vi "FP handling.vi"(6 "Set Modal?":bool, 7 "Mode":T3=enum."Restore Properties", 8 "error in (no error)":errorcluster, 10 "Properties Input":T1, 11 "VI in":refnum<vi>) -> (0 "error out":errorcluster, 2 "Retrieved Properties":T1, 3 "VI out":refnum<vi>)   [LabVIEW 2020]
uses:
  <vilib>/Utility/miscctls.llb/LVRectTypeDef.ctl
  FP UserInterface Properties--cluster.ctl
  FP handling mode selection--enum.ctl
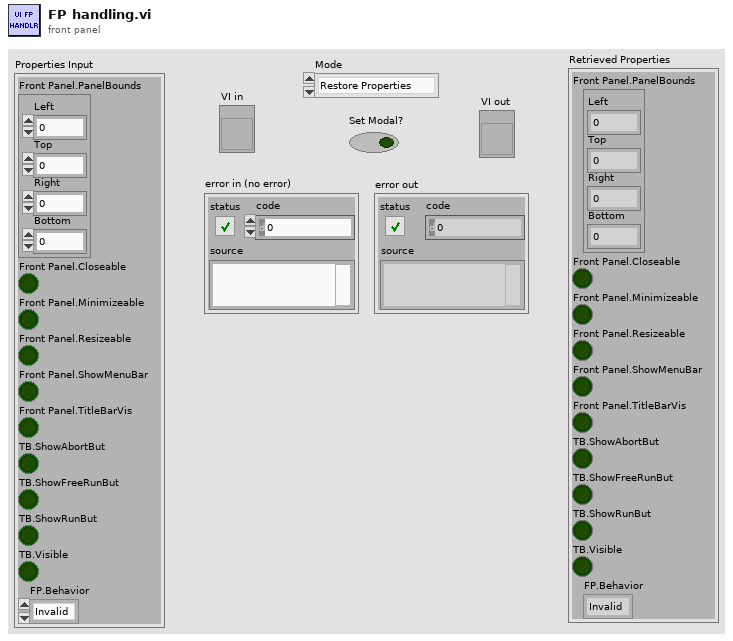
[diagram p1: front panel]
types:
  T1 = typedef "FP UserInterface Properties--cluster.ctl" = cluster{"Front Panel.PanelBounds":T2, "Front Panel.Closeable":bool, "Front Panel.Minimizeable":bool, "Front Panel.Resizeable":bool, "Front Panel.ShowMenuBar":bool, "Front Panel.TitleBarVis":bool, "TB.ShowAbortBut":bool, "TB.ShowFreeRunBut":bool, "TB.ShowRunBut":bool, "TB.Visible":bool, "FP.Behavior":enum32{"Invalid", "Default", "Floating", "Floating/Auto-Hide", "Modal"}}
  T2 = typedef "LVRectTypeDef.ctl" = cluster{"Left":i16, "Top":i16, "Right":i16, "Bottom":i16}
  T3 = typedef "FP handling mode selection--enum.ctl" = enum16{"Get Properties", "Restore Properties", "Set Full TouchScreen", "Properties Input"}
  T4 = enum32{"Invalid", "Default", "Floating", "Floating/Auto-Hide", "Modal"}
  T5 = cluster{"Front Panel Window:Panel Bounds":T2, "Front Panel.Closeable":bool, "Front Panel.Closeable":bool, "Front Panel.Closeable":bool, "Front Panel.Closeable":bool, "Front Panel.Closeable":bool, "Front Panel.Closeable":bool, "Front Panel.Closeable":bool, "Front Panel.Closeable":bool, "Front Panel.Closeable":bool, "Front Panel Window:Behavior":enum32{"Invalid", "Default", "Floating", "Floating/Auto-Hide", "Modal"}}
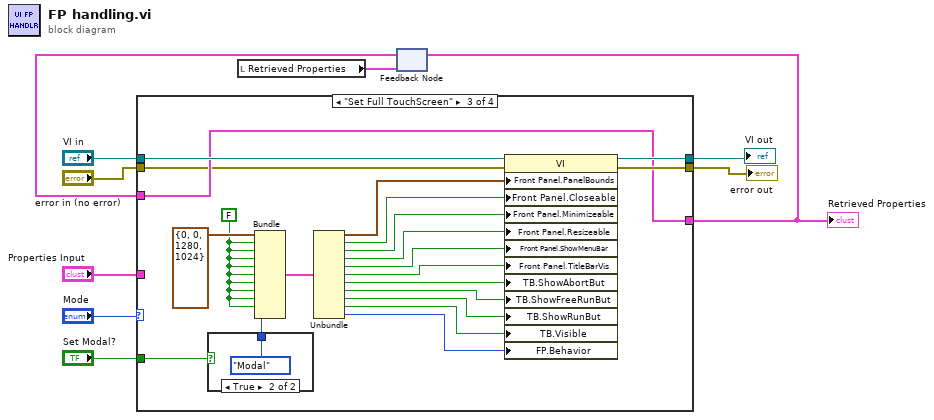
[diagram p0: block diagram]
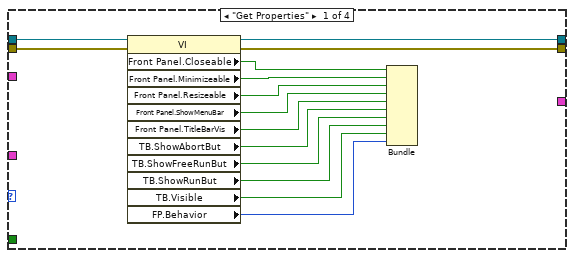
[diagram p2: hidden frame]
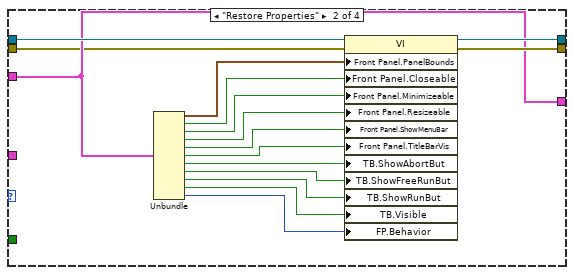
[diagram p3: hidden frame]
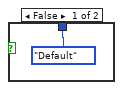
[diagram p4: hidden frame]
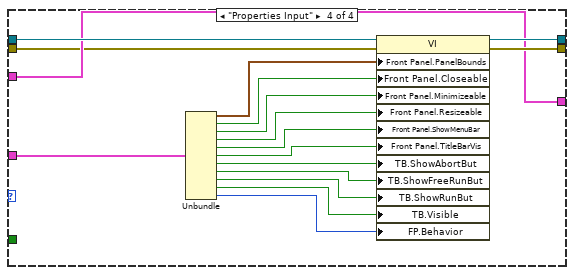
[diagram p5: hidden frame]
diagram:
  n1 = local read "Retrieved Properties"() -> (w3:T1)
  n2 = feedback #1(w3) -> (w6:T1)
  n3 = case shown="\"Set Full TouchScreen\"" "Mode" {
    tunnel: "VI in" -> [w14 w28 w49 w68]
    tunnel: [w13 w27 w48 w67] -> w8
    tunnel: [w12 w29 w50 w69] -> w9
    tunnel: [_ w26 w47 w66] -> w7
    tunnel: w6 -> [_ w26 w47 w66]
    tunnel: "error in (no error)" -> [w11 w25 w46 w65]
    tunnel: "Set Modal?" -> [_ _ w41 _]
    tunnel: "Properties Input" -> [_ _ _ w64]
    frame "Get Properties" {
      n4 = property class="VI"(reference=w14, error in=w11) -> (reference out=w12:refnum<vi>, error out=w13:errorcluster, "Front Panel.Closeable"=w22:bool, "Front Panel.Minimizeable"=w15:bool, "Front Panel.Resizeable"=w16:bool, "Front Panel.ShowMenuBar"=w17:bool, "Front Panel.TitleBarVis"=w18:bool, "TB.ShowAbortBut"=w19:bool, "TB.ShowFreeRunBut"=w20:bool, "TB.ShowRunBut"=w24:bool, "TB.Visible"=w21:bool, "FP.Behavior"=w23:T4)
      n5 = Bundle("Front Panel.Closeable"=w22, "Front Panel.Minimizeable"=w15, "Front Panel.Resizeable"=w16, "Front Panel.ShowMenuBar"=w17, "Front Panel.TitleBarVis"=w18, "TB.ShowAbortBut"=w19, "TB.ShowFreeRunBut"=w20, "TB.ShowRunBut"=w24, "TB.Visible"=w21, "FP.Behavior"=w23) -> ()  [unwired: 1 in, 1 out]
    }
    frame "Restore Properties" {
      n6 = Unbundle(w26) -> ("Front Panel.PanelBounds"=w30:T2, "Front Panel.Closeable"=w31:bool, "Front Panel.Minimizeable"=w32:bool, "Front Panel.Resizeable"=w33:bool, "Front Panel.ShowMenuBar"=w34:bool, "Front Panel.TitleBarVis"=w35:bool, "TB.ShowAbortBut"=w36:bool, "TB.ShowFreeRunBut"=w37:bool, "TB.ShowRunBut"=w38:bool, "TB.Visible"=w39:bool, "FP.Behavior"=w40:T4)
      n7 = property class="VI"(reference=w28, error in=w25, "Front Panel.PanelBounds"=w30, "Front Panel.Closeable"=w31, "Front Panel.Minimizeable"=w32, "Front Panel.Resizeable"=w33, "Front Panel.ShowMenuBar"=w34, "Front Panel.TitleBarVis"=w35, "TB.ShowAbortBut"=w36, "TB.ShowFreeRunBut"=w37, "TB.ShowRunBut"=w38, "TB.Visible"=w39, "FP.Behavior"=w40) -> (reference out=w29:refnum<vi>, error out=w27:errorcluster)
    }
    frame "Set Full TouchScreen" {
      w44 = FALSE ("Front Panel.Closeable")
      n8 = case shown="True" w41 {
        tunnel: [T4."Default" ("Front Panel Window:Behavior") T4."Modal" ("Front Panel Window:Behavior")] -> w43
        frame False {
        }
        frame True {
        }
      }
      n9 = Bundle("Front Panel Window:Panel Bounds"=T2 {"Left"=0, "Top"=0, "Right"=1280, "Bottom"=1024}, "Front Panel.Closeable"=w44, "Front Panel.Closeable"=w44, "Front Panel.Closeable"=w44, "Front Panel.Closeable"=w44, "Front Panel.Closeable"=w44, "Front Panel.Closeable"=w44, "Front Panel.Closeable"=w44, "Front Panel.Closeable"=w44, "Front Panel.Closeable"=w44, "Front Panel Window:Behavior"=w43) -> (w42:T5)  [unwired: 1 in]
      n10 = Unbundle(w42) -> ("Front Panel Window:Panel Bounds"=w51:T2, "Front Panel.Closeable"=w52:bool, "Front Panel.Closeable"=w53:bool, "Front Panel.Closeable"=w54:bool, "Front Panel.Closeable"=w55:bool, "Front Panel.Closeable"=w56:bool, "Front Panel.Closeable"=w57:bool, "Front Panel.Closeable"=w58:bool, "Front Panel.Closeable"=w59:bool, "Front Panel.Closeable"=w60:bool, "Front Panel Window:Behavior"=w61:T4)
      n11 = property class="VI"(reference=w49, error in=w46, "Front Panel.PanelBounds"=w51, "Front Panel.Closeable"=w52, "Front Panel.Minimizeable"=w53, "Front Panel.Resizeable"=w54, "Front Panel.ShowMenuBar"=w55, "Front Panel.TitleBarVis"=w56, "TB.ShowAbortBut"=w57, "TB.ShowFreeRunBut"=w58, "TB.ShowRunBut"=w59, "TB.Visible"=w60, "FP.Behavior"=w61) -> (reference out=w50:refnum<vi>, error out=w48:errorcluster)
    }
    frame "Properties Input" {
      n12 = Unbundle(w64) -> ("Front Panel.PanelBounds"=w70:T2, "Front Panel.Closeable"=w71:bool, "Front Panel.Minimizeable"=w72:bool, "Front Panel.Resizeable"=w73:bool, "Front Panel.ShowMenuBar"=w74:bool, "Front Panel.TitleBarVis"=w75:bool, "TB.ShowAbortBut"=w76:bool, "TB.ShowFreeRunBut"=w77:bool, "TB.ShowRunBut"=w78:bool, "TB.Visible"=w79:bool, "FP.Behavior"=w80:T4)
      n13 = property class="VI"(reference=w68, error in=w65, "Front Panel.PanelBounds"=w70, "Front Panel.Closeable"=w71, "Front Panel.Minimizeable"=w72, "Front Panel.Resizeable"=w73, "Front Panel.ShowMenuBar"=w74, "Front Panel.TitleBarVis"=w75, "TB.ShowAbortBut"=w76, "TB.ShowFreeRunBut"=w77, "TB.ShowRunBut"=w78, "TB.Visible"=w79, "FP.Behavior"=w80) -> (reference out=w69:refnum<vi>, error out=w67:errorcluster)
    }
  }
  "error out" <- w8
  "VI out" <- w9
  "Retrieved Properties" <- w7
  n14 = feedback-in #1(w7) -> ()
